vi "Transform3d_Times.vi"(9 "Scalar":dbl, 11 "in Transform3d":T1={"TRANSLATION3D"={"X"=0.0, "Y"=0.0, "Z"=0.0}, "ROTATION3D"={"Q_quaternion"={"R"=1.0, "V"=[0.0, 0.0, 0.0]}}} {"TRANSLATION3D"."Z" format="%14.3f"; "TRANSLATION3D"."Y" format="%14.3f"; "TRANSLATION3D"."X" format="%14.3f"}) -> (3 "Transform3d":T1={"TRANSLATION3D"={"X"=0.0, "Y"=0.0, "Z"=0.0}, "ROTATION3D"={"Q_quaternion"={"R"=1.0, "V"=[0.0, 0.0, 0.0]}}} {"TRANSLATION3D"."Z" format="%14.3f"; "TRANSLATION3D"."Y" format="%14.3f"; "TRANSLATION3D"."X" format="%14.3f"})   [LabVIEW 2019, in "Trajectory_Library.lvlib"]
doc: "Scales the transform by the scalar.\n\nParameters:\n - IN TRANSFORM - This TRANSFORM data structure\n - SCALAR - The scalar value to multiply the transform by\n\nResults:\n - OUT TRANSFORM - The multiplied transform data structure"
uses:
  Trajectory_Library.lvlib
  TRANSLATION3D.ctl
  QUATERNION.ctl
  ROTATION3D.ctl
  TRANSFORM3D.ctl
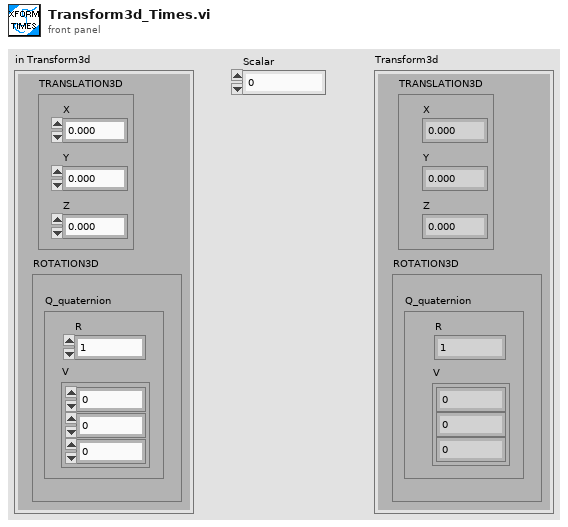
[diagram p1: front panel]
types:
  T1 = typedef "Trajectory_Library.lvlib/TRANSFORM3D.ctl" = cluster{"TRANSLATION3D":T2, "ROTATION3D":T3}
  T2 = typedef "Trajectory_Library.lvlib/TRANSLATION3D.ctl" = cluster{"X":dbl, "Y":dbl, "Z":dbl}
  T3 = typedef "Trajectory_Library.lvlib/ROTATION3D.ctl" = cluster{"Q_quaternion":T4}
  T4 = typedef "Trajectory_Library.lvlib/QUATERNION.ctl" = cluster{"R":dbl, "V":dbl[]}
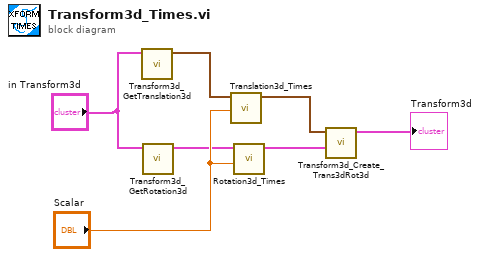
[diagram p0: block diagram]
diagram:
  n1 = call "Transform3d_GetTranslation3d.vi"("in Transform3d"="in Transform3d") -> ("Translation3d"=w2:T2)  [unwired: 10 in]
  n2 = call "Transform3d_GetRotation3d.vi"("in Transform3d"="in Transform3d") -> ("Rotation3d"=w1:T3)  [unwired: 10 in]
  n3 = call "Translation3d_Times.vi"("Scalar"="Scalar", "In Translation3d"=w2) -> ("Out Translation3d"=w3:T2)  [unwired: 9 in]
  n4 = call "Rotation3d_Times.vi"("Scalar"="Scalar", "in Rotation3d"=w1) -> ("out Rotation3d"=w4:T3)  [unwired: 9 in]
  n5 = call "Transform3d_Create_Trans3dRot3d.vi"("Rotation3d"=w4, "Translation3d"=w3) -> ("Transform3d"=→"Transform3d":T1)  [unwired: 9 in]
